vi "FieldDisp_Element_Rotate.vi"(9 "Angle":dbl, 11 "RotatedPictureInfo":T1) -> (3 "new picture":picture)   [LabVIEW 2019, in "Trajectory_Library.lvlib"]
doc: "Internal function -- should not be called directly by users.\n\nComplete documentation TBD."
uses:
  Trajectory_Library.lvlib
  TypeDef/FieldDisp_FieldElement.ctl
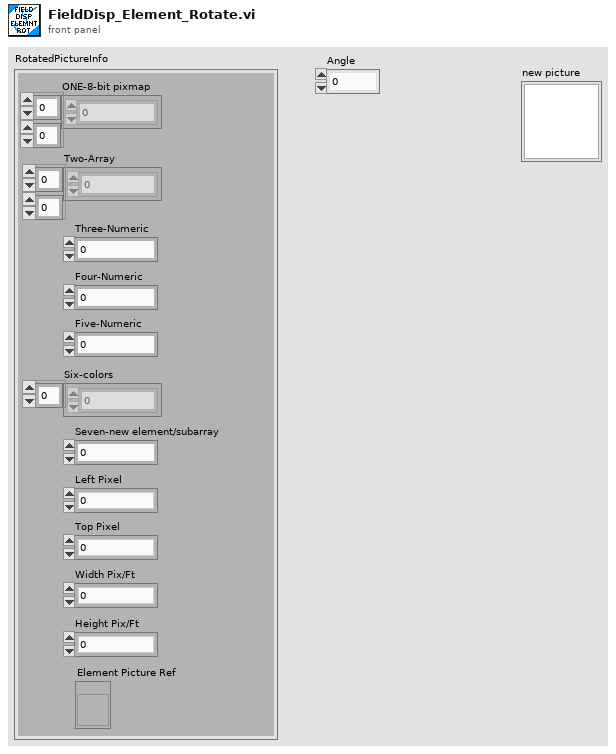
[diagram p1: front panel]
types:
  T1 = typedef "Trajectory_Library.lvlib/FieldDisp_FieldElement.ctl" = cluster{"ONE-8-bit pixmap":u8[][], "Two-Array":cdb[][], "Three-Numeric":i32, "Four-Numeric":i32, "Five-Numeric":cdb, "Six-colors":u32[], "Seven-new element/subarray":u32, "Left Pixel":dbl, "Top Pixel":dbl, "Width Pix/Ft":dbl, "Height Pix/Ft":dbl, "Element Picture Ref":refnum<vi>}
  T2 = typedef "imagedata.ctl" = cluster{"image type":i32, "image depth":i32, "image":u8[], "mask":u8[], "colors":u32[], "Rectangle":cluster{"left":i16, "top":i16, "right":i16, "bottom":i16}}
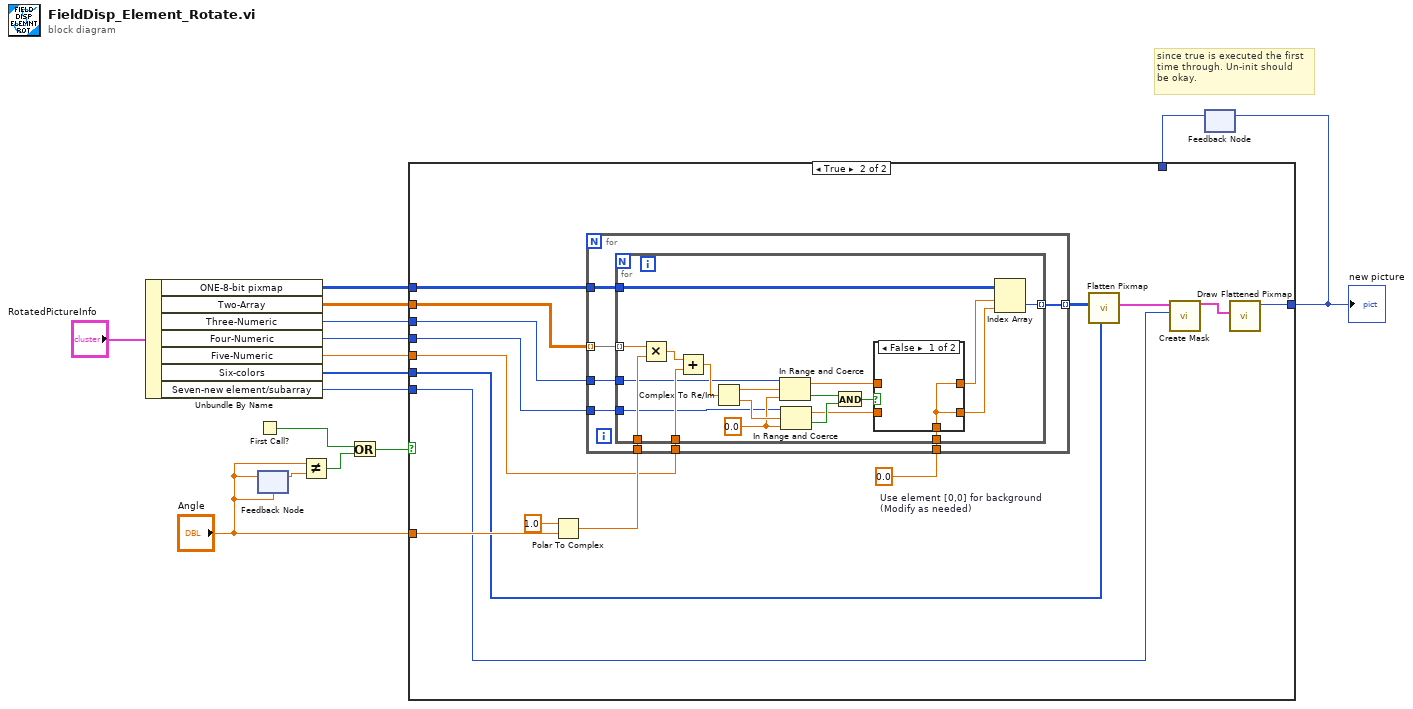
[diagram p0: block diagram]
diagram:
  # "since true is executed the first\ntime through. Un-init should\nbe okay."
  n1 = Unbundle By Name("RotatedPictureInfo") -> ("ONE-8-bit pixmap"=w14:u8[][], "Two-Array"=w13:cdb[][], "Three-Numeric"=w12:i32, "Four-Numeric"=w11:i32, "Five-Numeric"=w10:cdb, "Six-colors"=w9:u32[], "Seven-new element/subarray"=w8:u32)
  n2 = First Call?() -> (First Call?: T/F=w6:bool)
  n3 = feedback-in #1("Angle") -> ()
  n4 = feedback #1("Angle") -> (w1:dbl)
  n5 = Not Equal?(x="Angle", y=w1) -> (x != y?=w5:bool)
  n6 = Or(x=w6, y=w5) -> (x .or. y?=w7:bool)
  n7 = feedback #2() -> (w2:picture)  [unwired: 1 in]
  n8 = case shown="True" w7 {
    tunnel: "Angle" -> [_ w26]
    tunnel: [w16 w25] -> w3
    tunnel: w14 -> [_ w23]
    tunnel: w13 -> [_ w22]
    tunnel: w12 -> [_ w21]
    tunnel: w11 -> [_ w20]
    tunnel: w10 -> [_ w19]
    tunnel: w9 -> [_ w18]
    tunnel: w8 -> [_ w17]
    tunnel: w2 -> [w16 _]
    frame False {
    }
    frame True {
      w27 = 0.0  # Use element [0,0] for background (Modify as needed)
      n9 = Polar To Complex(1:w26, 2:1.0 ("r")) -> (0:w28:cdb)
      n10 = for {
        tunnel: w28 -> [w39]
        tunnel: w23 -> [w38]
        tunnel: w19 -> [w37]
        tunnel: w22 -> [w36] mode=indexing
        tunnel: [w35] -> w24 mode=indexing
        tunnel: w27 -> [w34]
        tunnel: w21 -> [w33]
        tunnel: w20 -> [w32]
        n11 = for {
          tunnel: w38 -> [w59]
          tunnel: w39 -> [w54]
          tunnel: [w58] -> w35 mode=indexing
          tunnel: w37 -> [w56]
          tunnel: w36 -> [w53] mode=indexing
          tunnel: w34 -> [w40]
          tunnel: w33 -> [w48]
          tunnel: w32 -> [w47]
          w49 = 0.0 ("lower limit")
          n12 = Multiply(x=w53, y=w54) -> (x*y=w55:cdb)
          n13 = Add(x=w55, y=w56) -> (x+y=w57:cdb)
          n14 = Complex To Re/Im(x + iy=w57) -> (x=w52:dbl, y=w51:dbl)
          n15 = In Range and Coerce(upper limit=w48, x=w52, lower limit=w49) -> (coerced(x)=w43:dbl, In Range?=w50:bool)
          n16 = In Range and Coerce(upper limit=w47, x=w51, lower limit=w49) -> (coerced(x)=w41:dbl, In Range?=w46:bool)
          n17 = And(x=w50, y=w46) -> (x .and. y?=w45:bool)
          n18 = case shown="False" w45 {
            tunnel: [w60 w62] -> w44
            tunnel: w43 -> [_ w62]
            tunnel: [w60 w61] -> w42
            tunnel: w41 -> [_ w61]
            tunnel: w40 -> [w60 _]
            frame False {
            }
            frame True {
            }
          }
          n19 = Index Array(array=w59, index (row)=w44, index (col)=w42) -> (element=w58:u8)
        }
      }
      n20 = call <vilib>:"Flatten Pixmap.vi"("colors"=w18, "8-bit pixmap"=w24) -> ("image data"=w30:T2)  [unwired: 9 in]
      n21 = call <vilib>:"Create Mask.vi"("Mask Color (Black)"=w17, "image data"=w30) -> ("image data"=w31:T2)  [unwired: 9 in]
      n22 = call <vilib>:"Draw Flattened Pixmap.vi"("image data"=w31) -> ("new picture"=w25:picture)  [unwired: 8 in]
    }
  }
  "new picture" <- w3
  n23 = feedback-in #2(w3) -> ()
